vi "Joint Reference Follower (MS IOP).vi"(7 "Offset Home2RCM [deg/mm]":dbl[](array[numeric])=[0.0, 0.0, 0.0, 0.0], 8 "PID Ctrl Cluster":T1={"L1 PID Gains"={"Kp"=0.005, "Kd"=0.5, "Ki"=0.0005}, "L2 PID Gains"={"Kp"=0.01, "Kd"=1.0, "Ki"=0.005}, "L3 PID Gains"={"Kp"=0.05, "Kd"=1.0, "Ki"=0.0005}, "L4 PID Gains"={"Kp"=0.1, "Kd"=0.1, "Ki"=0.0005}}, 9 "Ref Array [deg/mm]":dbl[](array[numeric])=[0.0, 0.0, 0.0, 0.0], 10 "error in":errorcluster, 11 "FPGA VI Reference In":refnum<k20>) -> (1 "Output Posit Array [deg/mm]":dbl[](array[numeric]), 2 "error out":errorcluster, 3 "FPGA VI Reference Out":refnum<k20>)   [LabVIEW 2016]
uses:
  <vilib>/rvi/errors/niLvFpgaAdjustHostInterfaceError.vi
  <vilib>/Utility/error.llb/Error Cluster From Error Code.vi
  Subsystems/Global Variables.vi
  <vilib>/rvi/interface/nirviReadWriteControl/nirviReadWriteControl.xnode
  FPGA Bitfiles/IRISSTrack_FPGATarget2_IRISSFPGAIORIO_4NTO9ubhv-c.lvbitx
  IRISS_FPGA_IO_RIO.vi
  Library/KevinLibraryAll/labview/KevLib01.lvlib
  NiFpgaLv.dll
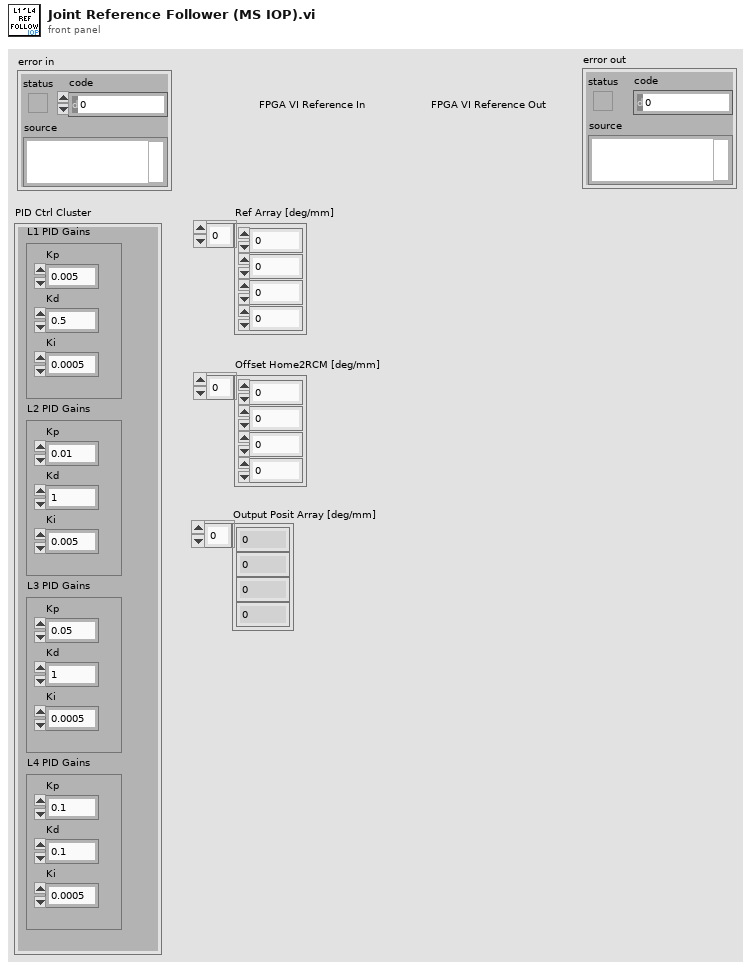
[diagram p1: front panel]
types:
  T1 = cluster{"L1 PID Gains":cluster{"Kp":dbl, "Kd":dbl, "Ki":dbl}, "L2 PID Gains":cluster{"Kp":dbl, "Kd":dbl, "Ki":dbl}, "L3 PID Gains":cluster{"Kp":dbl, "Kd":dbl, "Ki":dbl}, "L4 PID Gains":cluster{"Kp":dbl, "Kd":dbl, "Ki":dbl}}
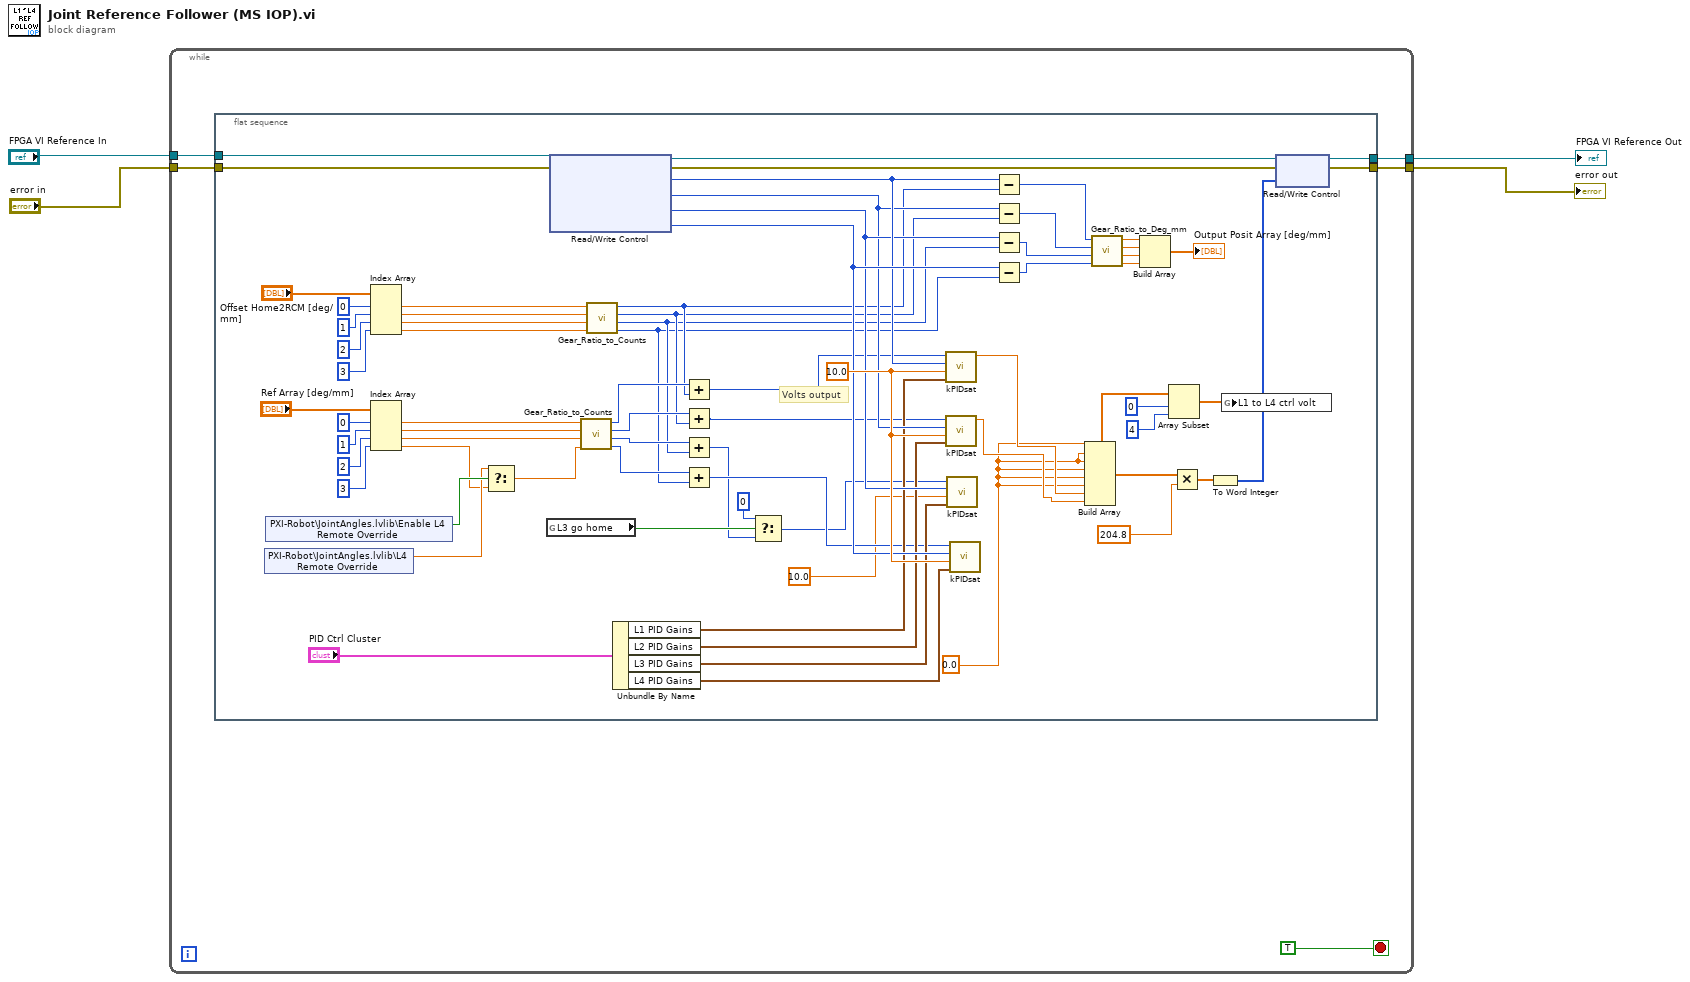
[diagram p0: block diagram]
diagram:
  n1 = while {
    tunnel: [w9] -> w1
    tunnel: [w8] -> w4
    tunnel: "FPGA VI Reference In" -> [w7]
    tunnel: "error in" -> [w6]
    stop <- TRUE ("Boolean") stop-if-true
    n2 = flat-sequence {
      tunnel: [w62] -> w9
      tunnel: [w61] -> w8
      tunnel: w7 -> [w43]
      tunnel: w6 -> [w42]
      frame #0 {
        w10 = 0.0 ("element")
        w67 = 10.0 ("Sat Limit")
        # "Volts output"
        n3 = shared-variable "PXI-Robot\\JointAngles.lvlib\\L4 Remote Override"() -> (w21:dbl)  [unwired: 1 in, 1 out]
        n4 = shared-variable "PXI-Robot\\JointAngles.lvlib\\Enable L4 Remote Override"() -> (w22:bool)  [unwired: 1 in, 1 out]
        n5 = Index Array(array="Offset Home2RCM [deg/mm]", index #1=0 ("index"), index #2=1 ("index"), index #3=2 ("index"), index #4=3 ("index")) -> (element #1=w41:dbl, element #2=w40:dbl, element #3=w39:dbl, element #4=w38:dbl)
        n6 = Index Array(array="Ref Array [deg/mm]", index #1=0 ("index"), index #2=1 ("index"), index #3=2 ("index"), index #4=3 ("index")) -> (element #1=w75:dbl, element #2=w74:dbl, element #3=w73:dbl, element #4=w20:dbl)
        n7 = Select(t=w21, s=w22, f=w20) -> (s? t:f=w19:dbl)
        n8 = global read "Global Variables.vi" "L3 go home"() -> (w26:bool)
        n9 = xnode "Read/Write Control"("FPGA VI Reference In"=w43, "error in"=w42) -> ("FPGA VI Reference Out"=w64:refnum<k20>, "error out"=w63:errorcluster, "32 bit Position 1"=w50:i32, "32 bit Position 3"=w48:i32, "32 bit Position C1-1"=w49:i32, "32 bit Position C1-4"=w59:i32)
        n10 = call "Gear_Ratio_to_Counts.vi"("theta 4"=w19, "theta 3"=w73, "theta 2"=w74, "theta 1"=w75) -> ("j4"=w31:i32, "j3"=w32:i32, "j2"=w33:i32, "j1"=w34:i32)
        n11 = call "Gear_Ratio_to_Counts.vi"("theta 4"=w38, "theta 3"=w39, "theta 2"=w40, "theta 1"=w41) -> ("j4"=w27:i32, "j3"=w28:i32, "j2"=w29:i32, "j1"=w30:i32)
        n12 = Unbundle By Name("PID Ctrl Cluster") -> ("L1 PID Gains"=w47:cluster{"Kp":dbl, "Kd":dbl, "Ki":dbl}, "L2 PID Gains"=w46:cluster{"Kp":dbl, "Kd":dbl, "Ki":dbl}, "L3 PID Gains"=w45:cluster{"Kp":dbl, "Kd":dbl, "Ki":dbl}, "L4 PID Gains"=w44:cluster{"Kp":dbl, "Kd":dbl, "Ki":dbl})
        n13 = Add(x=w34, y=w30) -> (x+y=w37:i32)
        n14 = Add(x=w33, y=w29) -> (x+y=w36:i32)
        n15 = Add(x=w32, y=w28) -> (x+y=w25:i32)
        n16 = Add(x=w31, y=w27) -> (x+y=w35:i32)
        n17 = Select(t=0 ("index"), s=w26, f=w25) -> (s? t:f=w23:i32)
        n18 = call "kPIDsat.vi"("PID Gains"=w47, "Sat Limit"=w67, "Position"=w50, "Reference"=w37) -> ("Control"=w12:dbl)  [unwired: 7 in]
        n19 = call "kPIDsat.vi"("PID Gains"=w46, "Sat Limit"=w67, "Position"=w48, "Reference"=w36) -> ("Control"=w11:dbl)  [unwired: 7 in]
        n20 = call "kPIDsat.vi"("PID Gains"=w45, "Sat Limit"=10.0, "Position"=w49, "Reference"=w23) -> ()  [unwired: 7 in, 1 out]
        n21 = call "kPIDsat.vi"("PID Gains"=w44, "Sat Limit"=w67, "Position"=w59, "Reference"=w35) -> ()  [unwired: 7 in, 1 out]
        n22 = Subtract(x=w50, y=w30) -> (x-y=w54:i32)
        n23 = Subtract(x=w48, y=w29) -> (x-y=w53:i32)
        n24 = Subtract(x=w49, y=w28) -> (x-y=w52:i32)
        n25 = Subtract(x=w59, y=w27) -> (x-y=w51:i32)
        n26 = Build Array(w10, w10, w10, w10, w10, w10, w12, w11) -> (w15:dbl[])
        n27 = call "Gear_Ratio_to_Deg_mm.vi"("j4"=w51, "j3"=w52, "j2"=w53, "j1"=w54) -> ("theta 4"=w55:dbl, "theta 3"=w56:dbl, "theta 2"=w57:dbl, "theta 1"=w58:dbl)
        n28 = Build Array(w58, w57, w56, w55) -> (→"Output Posit Array [deg/mm]":dbl[])
        n29 = Array Subset(array=w15, index=0, length=4) -> (w16:dbl[])
        n30 = Multiply(x=w15, y=204.8) -> (x*y=w66:dbl[])
        n31 = To Word Integer(number=w66) -> (16bit integer=w65:i16[])
        n32 = global write "Global Variables.vi" "L1 to L4 ctrl volt"(w16) -> ()
        n33 = xnode "Read/Write Control"("FPGA VI Reference In"=w64, "error in"=w63, "AO"=w65) -> ("FPGA VI Reference Out"=w62:refnum<k20>, "error out"=w61:errorcluster)
      }
    }
  }
  "error out" <- w4
  "FPGA VI Reference Out" <- w1
